vi "FindFaces.vi"(7 "File Path":path, 8 "error in":errorcluster, 10 "Faces In":T2[](array[typedef]) {"Rotation" format="%.2f"; "Left" scale=0.0..1024.0; "Right" scale=0.0..1024.0}, 11 "Image In":T1) -> (0 "error out":errorcluster, 2 "Faces":T2[](array[typedef]) {"Rotation" format="%.2f"; "Left" scale=0.0..1024.0; "Right" scale=0.0..1024.0}, 3 "Array":T1[](array[typedef]))   [LabVIEW 2019]
uses:
  <vilib>/vision/Image Controls.llb/IMAQ Image.ctl
panel:
  out "Image out":T1
  in  "index":i32
  out "size(s)":i32
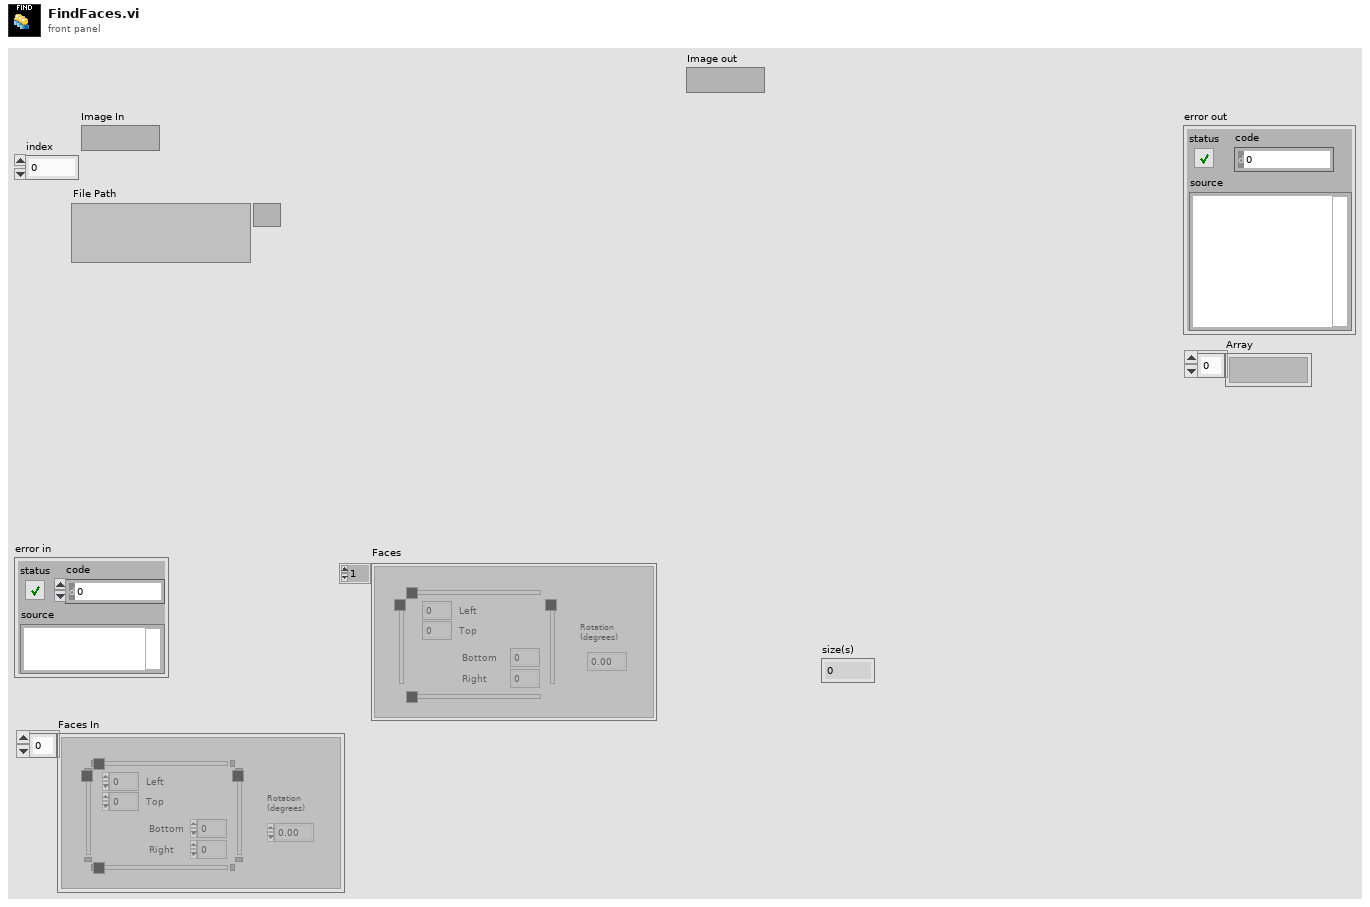
[diagram p1: front panel]
types:
  T1 = typedef "IMAQ Image.ctl" = refnum<image>
  T2 = typedef "IMAQ Rectangle" = cluster{"Left":i32, "Top":i32, "Right":i32, "Bottom":i32, "Rotation":dbl}
  T3 = typedef "Image Type" = u32
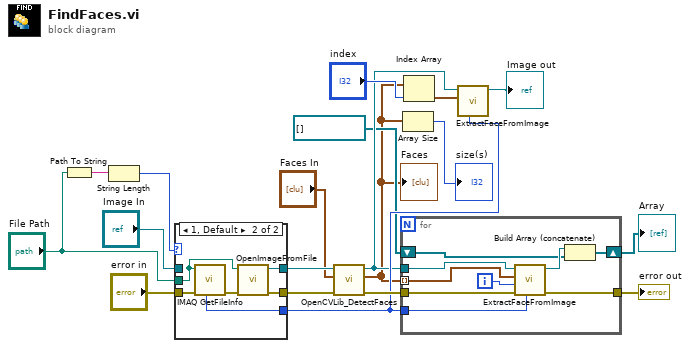
[diagram p0: block diagram]
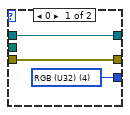
[diagram p2: hidden frame]
diagram:
  n1 = Path To String(path="File Path") -> (string=w5:string)
  n2 = String Length(string=w5) -> (length=w3:i32)
  n3 = case shown="1, Default" w3 {
    tunnel: "File Path" -> [_ w26]
    tunnel: [w21 w28] -> w19
    tunnel: [w20 w27] -> w18
    tunnel: [w22 w25] -> w9
    tunnel: "Image In" -> [w21 _]
    tunnel: "error in" -> [w20 w24]
    frame 0 {
      w22 = T3 4 items=["Grayscale (U8)", "Grayscale (I16)", "Grayscale (SGL)", "Complex (CSG)", "RGB (U32)", "HSL (U32)", "RGB (U64)", "Grayscale (U16)"] ("Image Type")
    }
    frame 1, Default {
      n4 = call "IMAQ GetFileInfo"("error in (no error)"=w24, "File Path"=w26) -> ("error out"=w23:errorcluster, "Image Type"=w25:T3)  [unwired: 8 out]
      n5 = call "OpenImageFromFile.vi"("error in (no error)"=w23, "File Path"=w26) -> ("error out"=w27:errorcluster, "Image"=w28:T1)  [unwired: 8 in]
    }
  }
  n6 = call "OpenCVLib_DetectFaces.vi"("error in (no error)"=w18, "Faces In"="Faces In", "Image Src"=w19) -> ("error out"=w13:errorcluster, "Faces"=w1:T2[], "Image Dst Out"=w7:T1)  [unwired: 6 in]
  "Faces" <- w1
  n7 = for {
    tunnel: w1 -> [w29] mode=indexing
    tunnel: w7 -> [w37]
    shift-right: [w34] -> w16
    shift-left: T1[] [] -> [w33]
    tunnel: w13 -> [w32]
    tunnel: [w31] -> w12
    tunnel: w9 -> [w30]
    i -> [w36]
    n8 = call "ExtractFaceFromImage.vi"("Image Type"=w30, "error in (no error)"=w32, "Numeric"=w36, "Rectangle"=w29, "Image in"=w37) -> ("error out"=w31:errorcluster, "Image out"=w35:T1)  [unwired: 5 in]
    n9 = Build Array (concatenate)(w35, w33) -> (w34:T1[])
  }
  "error out" <- w12
  "Array" <- w16
  n10 = Array Size(array=w1) -> (size(s)=→"size(s)":i32)
  n11 = Index Array(array=w1, index="index") -> (element=w8:T2)
  n12 = call "ExtractFaceFromImage.vi"("Image Type"=w9, "Rectangle"=w8, "Image in"=w7) -> ("Image out"=→"Image out":T1)  [unwired: 7 in, 1 out]
